vi "Add circle to list.vi"(4 "neighbor circle ? (N)":bool, 6 "circle in circle ? (N)":bool, 7 "neighbor distance":dbl=1.0 format="%.2f", 10 "circle":cluster{"x":i16, "y":i16, "radius":i32}, 11 "circle list":cluster{"x":i16, "y":i16, "radius":i32}[](array[cluster])) -> (3 "circle list out":cluster{"x":i16, "y":i16, "radius":i32}[](array[cluster]))   [LabVIEW 2017]
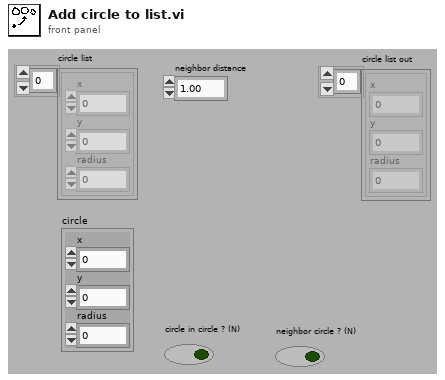
[diagram p1: front panel]
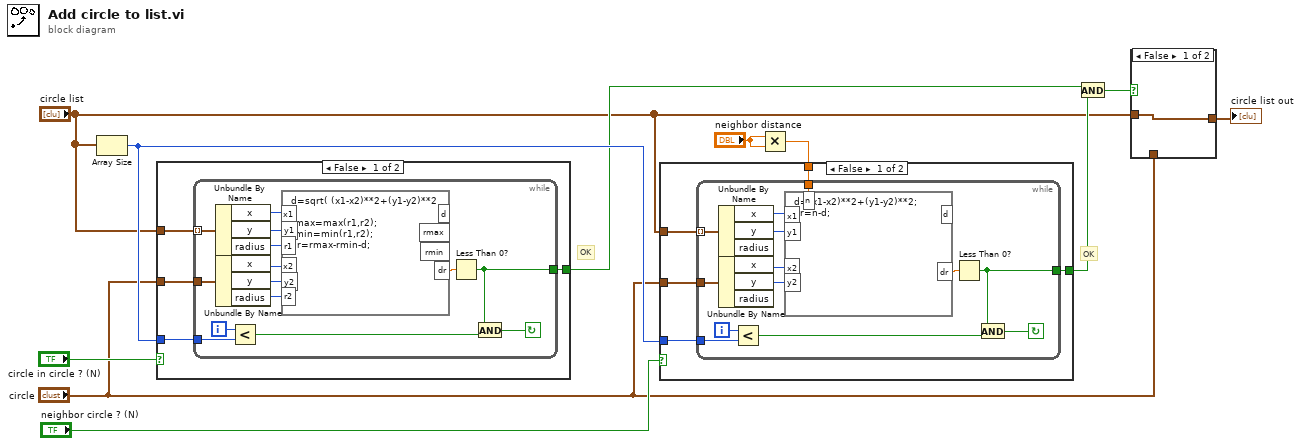
[diagram p0: block diagram]
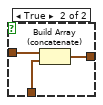
[diagram p2: hidden frame]
diagram:
  # "OK"
  # "OK"
  n1 = Array Size(array="circle list") -> (size(s)=w10:i32)
  n2 = case shown="False" "circle in circle ? (N)" {
    selector: "circle in circle ? (N)" -> [_ w30]
    tunnel: w10 -> [w15 _]
    tunnel: "circle list" -> [w14 _]
    tunnel: "circle" -> [w13 _]
    tunnel: [w12 w30] -> w5
    frame False {
      n3 = while {
        tunnel: [w16] -> w12
        tunnel: w13 -> [w24]
        tunnel: w14 -> [w25] mode=indexing
        tunnel: w15 -> [w28]
        i -> [w29]
        stop <- w26 continue-if-true
        n4 = Unbundle By Name(w25) -> ("x"=w22:i16, "y"=w21:i16, "radius"=w20:i32)
        n5 = Unbundle By Name(w24) -> ("x"=w19:i16, "y"=w17:i16, "radius"=w18:i32)
        n6 = Less?(x=w29, y=w28) -> (x < y?=w27:bool)
        n7 = formula code="d=sqrt( (x1-x2)**2+(y1-y2)**2 );\nrmax=max(r1,r2);\nrmin=min(r1,r2);\ndr=rmax-rmin-d;"("x1"=w22, "y1"=w21, "r1"=w20, "x2"=w19, "y2"=w17, "r2"=w18) -> ("dr"=w23:dbl)  [unwired: 3 out]
        n8 = Less Than 0?(x=w23) -> (x < 0?=w16:bool)
        n9 = And(x=w16, y=w27) -> (x .and. y?=w26:bool)
      }
    }
    frame True {
    }
  }
  n10 = Multiply(x="neighbor distance", y="neighbor distance") -> (x*y=w8:dbl)
  n11 = case shown="False" "neighbor circle ? (N)" {
    selector: "neighbor circle ? (N)" -> [_ w49]
    tunnel: w10 -> [w35 _]
    tunnel: "circle list" -> [w34 _]
    tunnel: "circle" -> [w33 _]
    tunnel: [w32 w49] -> w6
    tunnel: w8 -> [w31 _]
    frame False {
      n12 = while {
        tunnel: w31 -> [w36]
        tunnel: [w37] -> w32
        tunnel: w33 -> [w43]
        tunnel: w34 -> [w44] mode=indexing
        tunnel: w35 -> [w47]
        i -> [w48]
        stop <- w45 continue-if-true
        n13 = Unbundle By Name(w44) -> ("x"=w41:i16, "y"=w40:i16)  [unwired: 1 out]
        n14 = Unbundle By Name(w43) -> ("x"=w39:i16, "y"=w38:i16)  [unwired: 1 out]
        n15 = Less?(x=w48, y=w47) -> (x < y?=w46:bool)
        n16 = formula code="d=(x1-x2)**2+(y1-y2)**2;\ndr=n-d;"("x1"=w41, "y1"=w40, "x2"=w39, "y2"=w38, "n"=w36) -> ("dr"=w42:dbl)  [unwired: 1 out]
        n17 = Less Than 0?(x=w42) -> (x < 0?=w37:bool)
        n18 = And(x=w37, y=w46) -> (x .and. y?=w45:bool)
      }
    }
    frame True {
    }
  }
  n19 = And(x=w5, y=w6) -> (x .and. y?=w4:bool)
  n20 = case shown="False" w4 {
    tunnel: "circle list" -> [w50 w53]
    tunnel: [w50 w52] -> w2
    tunnel: "circle" -> [_ w51]
    frame False {
    }
    frame True {
      n21 = Build Array (concatenate)(w53, w51) -> (w52:cluster{"x":i16, "y":i16, "radius":i32}[])
    }
  }
  "circle list out" <- w2
